vi "Rodrigues (RMat To RVec).vi"(8 "error in (no error)":errorcluster, 11 "Rotation Matrix":T1=[[1.0, 0.0, 0.0], [0.0, 1.0, 0.0], [0.0, 0.0, 1.0]]) -> (0 "error out":errorcluster, 3 "rvec":T2)   [LabVIEW 2020, in "g_ar_toolkit.ar.lvlib"]
uses:
  g_ar_toolkit.ar.lvlib
  rvec.ctl
  <vilib>/Analysis/Matrix/Datatypes/RealMatrix.ctl
  g_ar_toolkit.common/g_ar_toolkit.common.lvlib
  <vilib>/Analysis/Matrix/NI_Matrix.lvlib
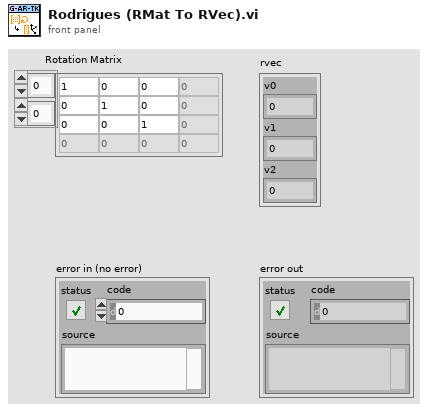
[diagram p1: front panel]
types:
  T1 = typedef "NI_Matrix.lvlib/RealMatrix.ctl" = dbl[][]
  T2 = typedef "g_ar_toolkit.ar.lvlib/rvec.ctl" = cluster{"v0":dbl, "v1":dbl, "v2":dbl}
  T3 = cluster{"Rotation Matrix[0]":dbl, "Rotation Matrix[1]":dbl, "Rotation Matrix[2]":dbl, "Rotation Matrix[3]":dbl, "Rotation Matrix[4]":dbl, "Rotation Matrix[5]":dbl, "Rotation Matrix[6]":dbl, "Rotation Matrix[7]":dbl, "Rotation Matrix[8]":dbl}
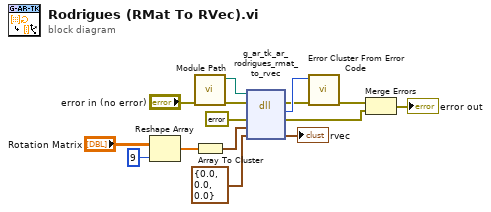
[diagram p0: block diagram]
diagram:
  n1 = Reshape Array("Rotation Matrix", 9 ("dimension size")) -> (w6:dbl[])
  n2 = call "Module Path.vi"("error in (no error)"="error in (no error)") -> ("error out"=w2:errorcluster, "Path"=w1:path)  [unwired: 9 in]
  n3 = Array To Cluster(array=w6) -> (cluster=w5:T3)
  n4 = dll-call lib="?" fn="g_ar_tk_ar_rodrigues_rmat_to_rvec" ("g_ar_toolkit.*.*:g_ar_tk_image_copy")(path in=w1, error in=w2, "error_cluster"=errorcluster {"status"=FALSE, "code"=0, "source"=""} ("error constant"), "rvec"=w5, "rmat"=T2 {"v0"=0.0, "v1"=0.0, "v2"=0.0} ("rvec")) -> (error out=w10:errorcluster, "MgErr"=w11:i32, "error_cluster"=w14:errorcluster, "rmat"=→"rvec":T2)  [unwired: 2 in, 1 out]
  n5 = call <vilib>:"Error Cluster From Error Code.vi"("error in (no error)"=w10, "error code (0)"=w11) -> ("error out"=w12:errorcluster)  [unwired: 7 in]
  n6 = Merge Errors(w12, w14) -> (→"error out":errorcluster)
